vi "Decode PicoHarp TT Data.vi"(8 "oflcorr_in":u64, 11 "rawbits":u32) -> (0 "oflcorr_out":u64, 1 "channel":u8, 3 "truetime":u64, 4 "markercode":u32)   [LabVIEW 2021, in "PTU Files.lvlib"]
uses:
  PTU Files.lvlib
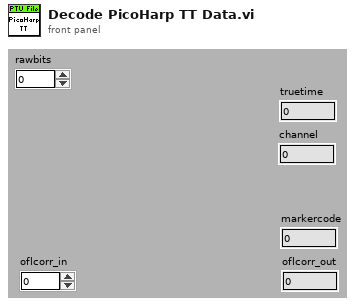
[diagram p1: front panel]
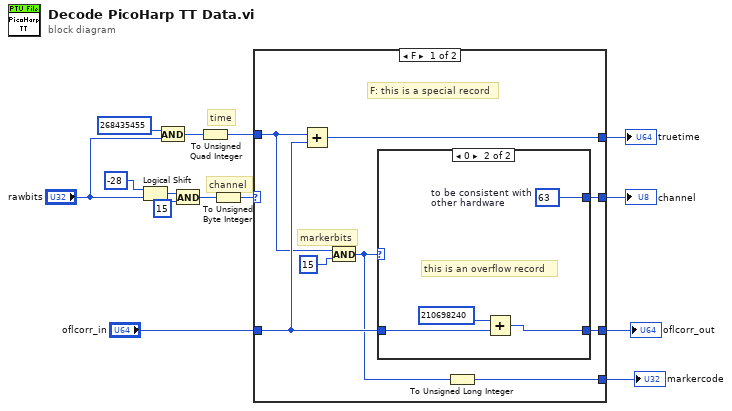
[diagram p0: block diagram]
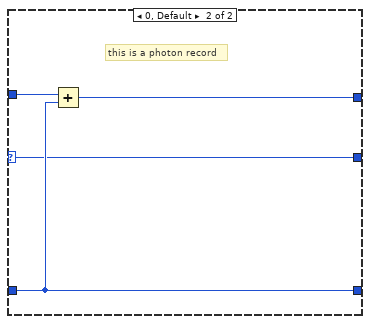
[diagram p3: hidden frame]
diagram:
  # "channel"
  # "time"
  n1 = Logical Shift(y=-28, x="rawbits") -> (x << y=w10:u32)
  n2 = And(x=u32 268435455, y="rawbits") -> (x .and. y?=w6:u32)
  n3 = And(x=w10, y=u32 15 ("x")) -> (x .and. y?=w13:u32)
  n4 = To Unsigned Quad Integer(1:w6) -> (0:w2:u64)
  n5 = To Unsigned Byte Integer(number=w13) -> (unsigned 8bit integer=w1:u8)
  n6 = case shown="F" w1 {
    selector: w1 -> [_ w28]
    tunnel: w2 -> [w19 w31]
    tunnel: "oflcorr_in" -> [w20 w29]
    tunnel: [w22 w29] -> w8
    tunnel: [w15 _] -> w9
    tunnel: [w18 w30] -> w12
    tunnel: [w16 w28] -> w14
    frame 15 {
      # "markerbits"
      # "F: this is a special record"
      n7 = Add(x=w19, y=w20) -> (x+y=w18:u64)
      n8 = And(x=w19, y=u64 15 ("x")) -> (x .and. y?=w17:u64)
      n9 = case shown="0" w17 {
        tunnel: w20 -> [w23 w27]
        tunnel: [w23 w26] -> w22
        tunnel: [_ w24] -> w16
        frame Default {
          # "this is a marker record"
        }
        frame 0 {
          w24 = u8 63  # to be consistent with other hardware
          # "this is an overflow record"
          n10 = Add(x=u64 210698240, y=w27) -> (x+y=w26:u64)
        }
      }
      n11 = To Unsigned Long Integer(number=w17) -> (unsigned 32bit integer=w15:u32)
    }
    frame 0, Default {
      # "this is a photon record"
      n12 = Add(x=w31, y=w29) -> (x+y=w30:u64)
    }
  }
  "channel" <- w14
  "truetime" <- w12
  "markercode" <- w9
  "oflcorr_out" <- w8
